vi "Create Evaluations.vi"(8 "error in (no error)":errorcluster, 11 "IEvaluation in":refnum<class "SpecAn_IM3.lvclass">) -> (0 "error out":errorcluster, 2 "Evaluations Out":T1[](array[typedef]) {"Low Limit" format="%#_13g"; "SI Scaling" items=["femto"=-15, "pico"=-12, "nano"=-9, "micro"=-6, "milli"=-3, "percent"=-2, ""=0, "kilo"=3, "mega"=6, "giga"=9, "tera"=12]}, 3 "IEvaluation out":refnum<class "SpecAn_IM3.lvclass">)   [LabVIEW 2018, in "SeqAuto Evaluations.lvlib" / "SpecAn_IM3.lvclass"]
uses:
  SpecAn_IM3.lvclass
  C:/Sequence Automation/Plugins/SeqAuto IEvaluation.lvlibp/SeqAuto IEvaluation.lvclass
  Plugins/TestStand API Tools (TSAT).lvlibp/Evaluation Actions/Includes/Controls/TSAT Evaluation.ctl
  Plugins/TestStand API Tools (TSAT).lvlibp/Evaluation Actions/Includes/Controls/TSAT Eval SI Unit Scaling.ctl
  Plugins/TestStand API Tools (TSAT).lvlibp/Evaluation Actions/Includes/Controls/TSAT Evaluation Type.ctl
  SpecAn_IM3.lvclass/SpecAn_IM3.ctl
  Read SA Pin.vi
  Plugins/SeqAuto IEvaluation.lvlibp/Read Measurement Name.vi
  Plugins/TestStand API Tools (TSAT).lvlibp/Evaluation Actions/TSAT Evaluation Actions.lvlib
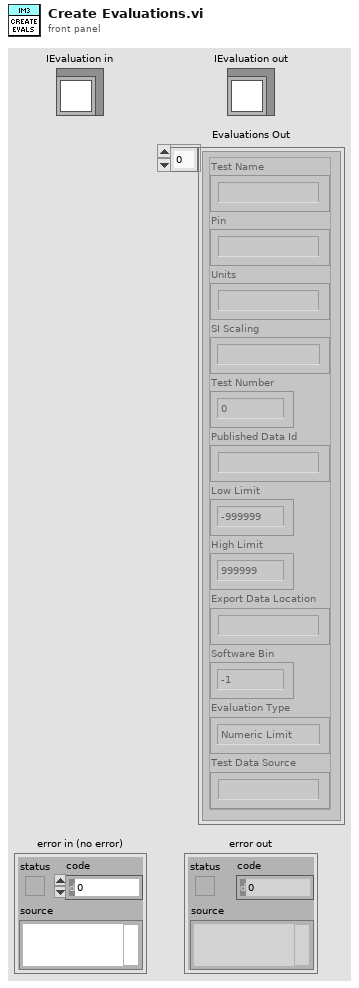
[diagram p1: front panel]
types:
  T1 = typedef "TestStand API Tools (TSAT).lvlibp/TSAT Evaluation Actions.lvlib/TSAT Evaluation.ctl" = cluster{"Test Name":string, "Pin":string, "Units":string, "SI Scaling":T2, "Test Number":i32, "Published Data Id":string, "Low Limit":dbl, "High Limit":dbl, "Export Data Location":string, "Software Bin":i64, "Evaluation Type":T3, "Test Data Source":string}
  T2 = typedef "TestStand API Tools (TSAT).lvlibp/TSAT Evaluation Actions.lvlib/TSAT Eval SI Unit Scaling.ctl" = i16
  T3 = typedef "TestStand API Tools (TSAT).lvlibp/TSAT Evaluation Actions.lvlib/TSAT Evaluation Type.ctl" = enum16{"Numeric Limit", "Pass/Fail", "None"}
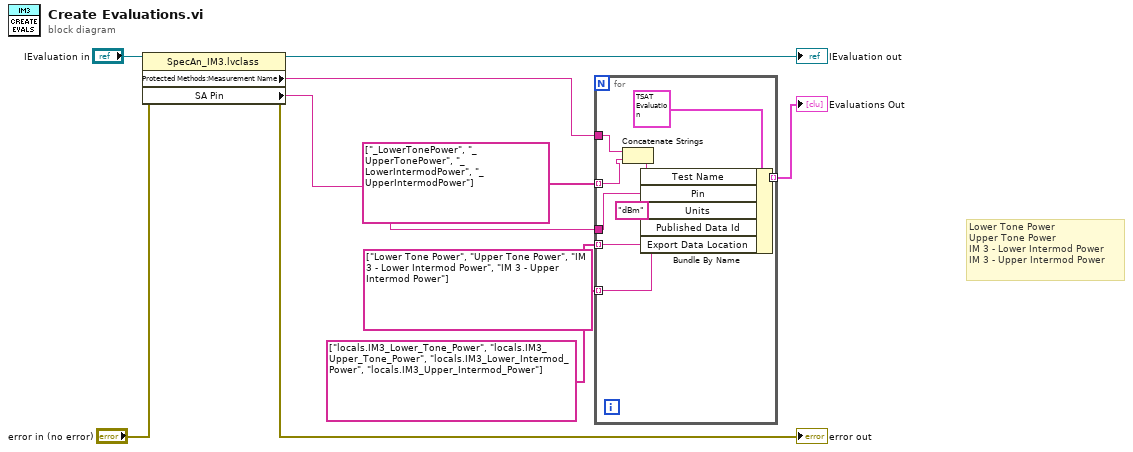
[diagram p0: block diagram]
diagram:
  # "Lower Tone Power\nUpper Tone Power\nIM 3 - Lower Intermod Power\nIM 3 - Upper Intermod Power"
  n1 = property class="SpecAn_IM3.lvclass"(reference="IEvaluation in", error in="error in (no error)") -> (reference out=→"IEvaluation out":refnum<class "SpecAn_IM3.lvclass">, error out=→"error out":errorcluster, "Protected Methods:Measurement Name"=w5:string, "SA Pin"=w3:string)
  n2 = for {
    tunnel: [w18] -> w6 mode=indexing
    tunnel: w5 -> [w16]
    tunnel: string[] ["_LowerTonePower", "_UpperTonePower", "_LowerIntermodPower", "_UpperIntermodPower"] -> [w15] mode=indexing
    tunnel: w3 -> [w13]
    tunnel: string[] ["Lower Tone Power", "Upper Tone Power", "IM 3 - Lower Intermod Power", "IM 3 - Upper Intermod Power"] -> [w12] mode=indexing
    tunnel: string[] ["locals.IM3_Lower_Tone_Power", "locals.IM3_Upper_Tone_Power", "locals.IM3_Lower_Intermod_Power", "locals.IM3_Upper_Intermod_Power"] -> [w11] mode=indexing
    n3 = Concatenate Strings(w16, w15) -> (w14:string)
    n4 = Bundle By Name(cluster=T1 {"Test Name"="", "Pin"="", "Units"="", "SI Scaling"=0, "Test Number"=0, "Published Data Id"="", "Low Limit"=-999999.0, "High Limit"=999999.0, "Export Data Location"="", "Software Bin"=-1, "Evaluation Type"=enum."Numeric Limit", "Test Data Source"=""} ("Evaluation"), "Test Name"=w14, "Pin"=w13, "Units"="dBm", "Published Data Id"=w12, "Export Data Location"=w11) -> (w18:T1)
  }
  "Evaluations Out" <- w6
